vi "Untitled 1.vi"() -> ()   [LabVIEW 2018]
panel:
  out "Root 2":dbl
  out "Root 1":dbl
  out "Has 1 root.":bool
  in  "Variable k":dbl
  out "Descriminant":dbl
  in  "Variable j":dbl
  in  "Variable i":dbl
  out "Hypotenous":dbl
  in  "Variable b":dbl
  in  "Variable a":dbl
  out "Is C > D":bool
  in  "Variable D":dbl
  in  "Variable C":dbl
  out "A + B =":dbl
  in  "Variable B":dbl
  in  "Variable A":dbl
  out "Full Name":string
  in  "Last Name":string
  in  "First Name":string
  # "i*x^2+j*x+k = 0"
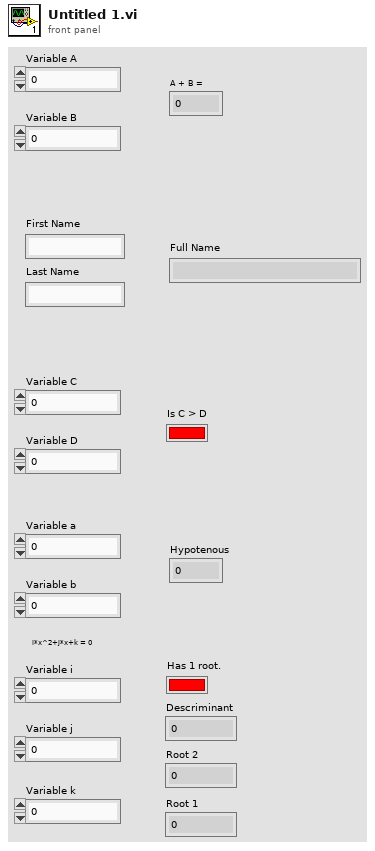
[diagram p1: front panel]
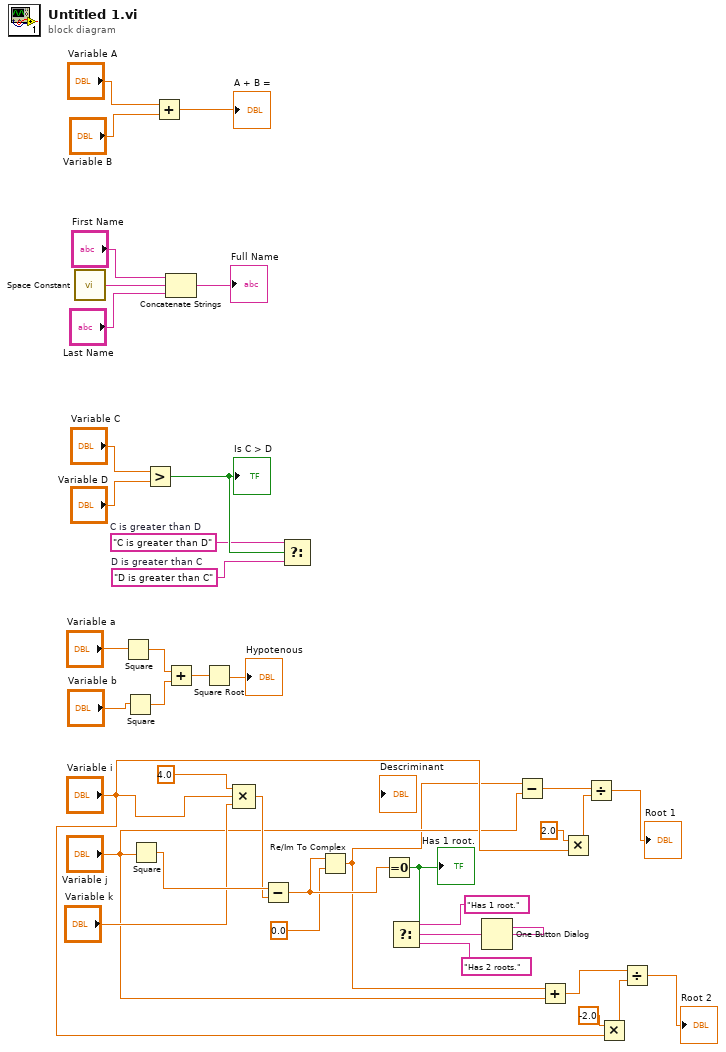
[diagram p0: block diagram]
diagram:
  w28 = "D is greater than C"  # D is greater than C
  w29 = "C is greater than D"  # C is greater than D
  n1 = call <vilib>:"Space Constant.vi"() -> ("String"=w37:string)
  n2 = Square(x="Variable a") -> (x^2=w24:dbl)
  n3 = Square(x="Variable b") -> (x^2=w27:dbl)
  n4 = Square(x="Variable j") -> (x^2=w21:dbl)
  n5 = Greater?(x="Variable C", y="Variable D") -> (0:w30:bool)
  "Is C > D" <- w30
  n6 = Add(x="Variable A", y="Variable B") -> (x+y=→"A + B =":dbl)
  n7 = Concatenate Strings "Concatenate Strings"("First Name", w37, "Last Name") -> (→"Full Name":string)
  n8 = Add(x=w24, y=w27) -> (x+y=w26:dbl)
  n9 = Square Root(x=w26) -> (sqrt(x)=→"Hypotenous":dbl)
  n10 = Compound Arithmetic op=MULTIPLY(4.0, "Variable i", "Variable k") -> (w18:dbl)
  n11 = Subtract(x=w21, y=w18) -> (x-y=w3:dbl)
  n12 = Select(t=w29, s=w30, f=w28) -> ()  [unwired: 1 out]
  n13 = Re/Im To Complex(1:0.0, 2:w3) -> (0:w1:cdb)
  n14 = Equal To 0?(x=w3) -> (x = 0?=w14:bool)
  "Has 1 root." <- w14
  n15 = Select(t="Has 1 root.", s=w14, f="Has 2 roots.") -> (s? t:f=w15:string)
  n16 = One Button Dialog(message=w15) -> ()  [unwired: 1 in, 1 out]
  n17 = Subtract(x=w1, y="Variable j") -> (x-y=w13:cdb)
  n18 = Add(x=w1, y="Variable j") -> (x+y=w5:cdb)
  n19 = Multiply(x=2.0, y="Variable i") -> (x*y=w11:dbl)
  n20 = Divide(x=w13, y=w11) -> (x/y=→"Root 1":cdb)
  n21 = Multiply(x=-2.0, y="Variable i") -> (x*y=w8:dbl)
  n22 = Divide(x=w5, y=w8) -> (x/y=→"Root 2":cdb)
